vi "CSP_saveFilter.vi"(8 "error in":errorcluster, 9 "File name":string="CSPFilter.bin", 11 "CSP.lvclass in":refnum<class "CSP.lvclass">) -> (0 "error out":errorcluster, 3 "CSP.lvclass out":refnum<class "CSP.lvclass">)   [LabVIEW 2016, in "Spatial Pattern Filter.lvlib" / "CSP.lvclass"]
uses:
  CSP.lvclass
  <vilib>/Analysis/Matrix/Datatypes/RealMatrix.ctl
  CSP.lvclass/CSP.ctl
  <vilib>/Analysis/Matrix/Comparison/Equal/Equal - RM,RM.vi
  <vilib>/Analysis/Matrix/NI_Matrix.lvlib
panel:
  # "This VI is a part of BCI Design library, http://www.ru-bci.org \nCopyright © 2020, Sotnikov Peter, All rights reserved. License: GNU GPLv3"
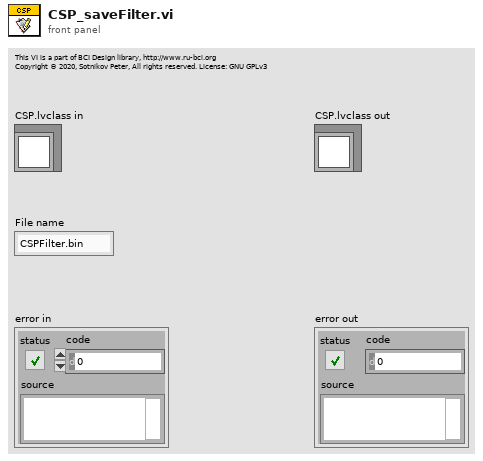
[diagram p1: front panel]
types:
  T1 = enum16{"big-endian, network order", "native, host order", "little-endian"}
  T2 = typedef "NI_Matrix.lvlib/RealMatrix.ctl" = dbl[][]
  T3 = cluster{"CSPMatrix":T2, "CovarianceMatrix1":T2, "CovarianceMatrix2":T2}[]
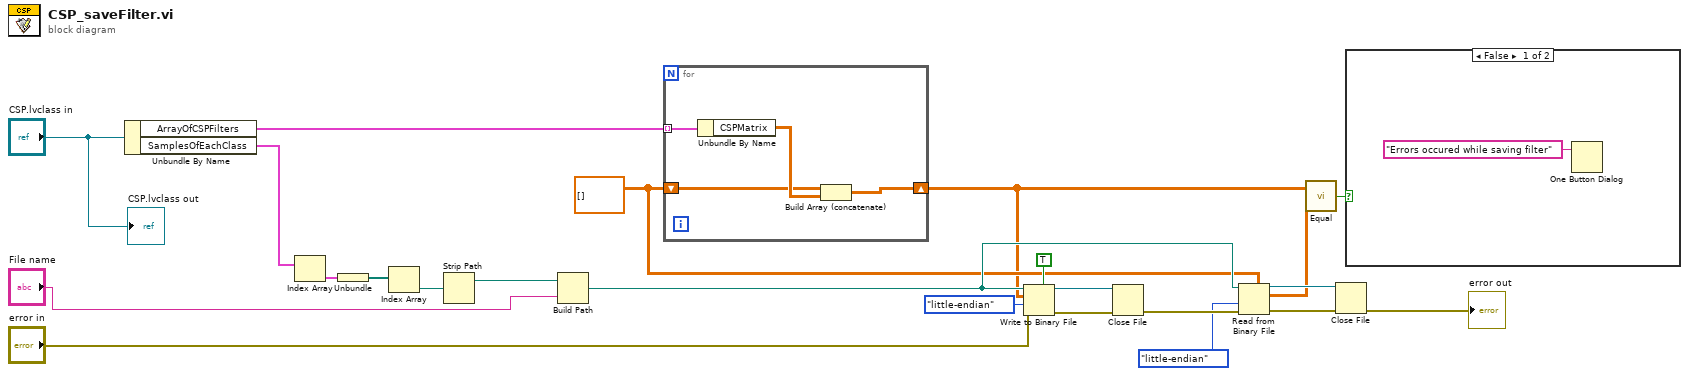
[diagram p0: block diagram]
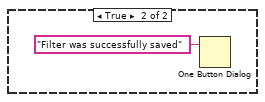
[diagram p2: hidden frame]
diagram:
  w11 = T2 [] ("CSPMatrix")
  n1 = Unbundle By Name("CSP.lvclass in") -> ("ArrayOfCSPFilters"=w20:T3, "SamplesOfEachClass"=w22:cluster{"ArrayOfFiles":path[]}[])
  n2 = Index Array(array=w22) -> (element=w3:cluster{"ArrayOfFiles":path[]})  [unwired: 1 in]
  n3 = Unbundle(w3) -> ("ArrayOfFiles"=w2:path[])
  n4 = Index Array(array=w2) -> (element=w1:path)  [unwired: 1 in]
  n5 = Strip Path(path=w1) -> (stripped path=w21:path)  [unwired: 1 out]
  n6 = Build Path(base path=w21, name or relative path="File name") -> (appended path=w13:path)
  n7 = for {
    tunnel: w20 -> [w27] mode=indexing
    shift-right: [w26] -> w7
    shift-left: w11 -> [w24]
    n8 = Unbundle By Name(w27) -> ("CSPMatrix"=w25:T2)
    n9 = Build Array (concatenate)(w24, w25) -> (w26:T2)
  }
  n10 = Write to Binary File(file (use dialog)=w13, data=w7, error in="error in", 5:TRUE ("prepend array or string size? (T)"), 9:T1."little-endian" ("byte order (0:big-endian, network order)")) -> (refnum out=w16:refnum<file>, error out=w15:errorcluster)  [unwired: 1 in, 1 out]
  n11 = Close File(refnum=w16, error in=w15) -> (error out=w14:errorcluster)  [unwired: 1 out]
  n12 = Read from Binary File(5:w11, 8:w14, 9:T1."little-endian" ("byte order (0:big-endian, network order)"), 11:w13) -> (0:w10:errorcluster, 2:w6:T2, 3:w9:refnum<file>)  [unwired: 2 in, 1 out]
  n13 = call-poly <vilib>:"Equal.vi"("Real Matrix B"=w6, "Real Matrix A"=w7) -> ("A = B?"=w5:bool)
  n14 = Close File(refnum=w9, error in=w10) -> (error out=→"error out":errorcluster)  [unwired: 1 out]
  n15 = case shown="False" w5 {
    frame False {
      n16 = One Button Dialog(message="Errors occured while saving filter") -> ()  [unwired: 1 in, 1 out]
    }
    frame True {
      n17 = One Button Dialog(message="Filter was successfully saved") -> ()  [unwired: 1 in, 1 out]
    }
  }
  "CSP.lvclass out" <- "CSP.lvclass in"
